vi "Letter Check.vi"(11 "Letter_Ref":refnum<vi>) -> ()   [LabVIEW 2015]
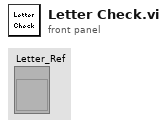
[diagram p1: front panel]
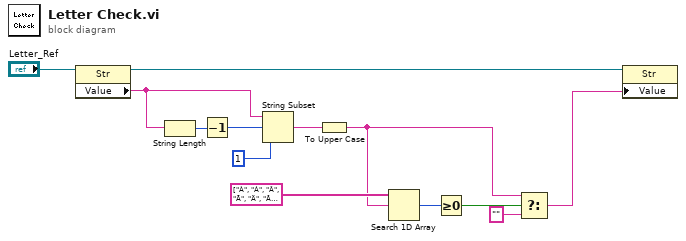
[diagram p0: block diagram]
diagram:
  n1 = property class="Str"(reference="Letter_Ref") -> (reference out=w9:refnum<vi>, "Value"=w1:string)  [unwired: 1 in, 1 out]
  n2 = String Length(string=w1) -> (length=w10:i32)
  n3 = Decrement(x=w10) -> (x-1=w11:i32)
  n4 = String Subset(string=w1, offset (0)=w11, length (rest)=1 ("length (rest)")) -> (substring=w13:string)
  n5 = To Upper Case(1:w13) -> (0:w4:string)
  n6 = Search 1D Array(1D array=string[] ["À", "Á", "Â", "Ã", "Ä", "Å", "Æ", "Ç", "È", "É", "Ê", "Ë", "Ì", "Í", "Î", "Ï", "Ð", "Ñ", "Ò", "Ó", "Ô", "Õ", "Ö", "×", "Ø", "Ù", "Ú", "Û", "Ü", "Ý", "Þ", "ß"] ("Letter"), element=w4) -> (index of element=w6:i32)  [unwired: 1 in]
  n7 = Greater Or Equal To 0?(x=w6) -> (x >= 0?=w5:bool)
  n8 = Select(t=w4, s=w5, f="") -> (s? t:f=w2:string)
  n9 = property class="Str"(reference=w9, "Value"=w2) -> ()  [unwired: 1 in, 2 out]
